vi "IMAQ FPGA Camera Link Acquisition.vi"   [LabVIEW 2017]
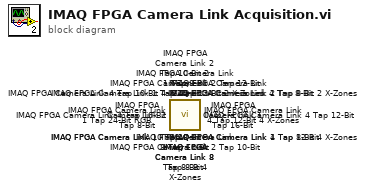
[diagram p0: block diagram]
diagram:
  n1 = call <vilib>:"IMAQ FPGA Camera Link 8 Tap 10-Bit.vi"() -> ()  [unwired: 8 in, 4 out]
  n2 = call <vilib>:"IMAQ FPGA Camera Link 2 Tap 12-Bit 2 X-Zones.vi"() -> ()  [unwired: 8 in, 4 out]
  n3 = call <vilib>:"IMAQ FPGA Camera Link 1 Tap 24-Bit RGB.vi"() -> ()  [unwired: 8 in, 4 out]
  n4 = call <vilib>:"IMAQ FPGA Camera Link 4 Tap 12-Bit 4 X-Zones.vi"() -> ()  [unwired: 8 in, 4 out]
  n5 = call <vilib>:"IMAQ FPGA Camera Link 4 Tap 10-Bit 4 X-Zones.vi"() -> ()  [unwired: 8 in, 4 out]
  n6 = call <vilib>:"IMAQ FPGA Camera Link 2 Tap 10-Bit 2 X-Zones.vi"() -> ()  [unwired: 8 in, 4 out]
  n7 = call <vilib>:"IMAQ FPGA Camera Link 8 Tap 8-Bit 4 X-Zones.vi"() -> ()  [unwired: 8 in, 4 out]
  n8 = call <vilib>:"IMAQ FPGA Camera Link 4 Tap 8-Bit 4 X-Zones.vi"() -> ()  [unwired: 8 in, 4 out]
  n9 = call <vilib>:"IMAQ FPGA Camera Link 10 Tap 8-Bit.vi"() -> ()  [unwired: 8 in, 4 out]
  n10 = call <vilib>:"IMAQ FPGA Camera Link 4 Tap 10-Bit.vi"() -> ()  [unwired: 8 in, 4 out]
  n11 = call <vilib>:"IMAQ FPGA Camera Link 4 Tap 12-Bit.vi"() -> ()  [unwired: 8 in, 4 out]
  n12 = call <vilib>:"IMAQ FPGA Camera Link 4 Tap 8-Bit.vi"() -> ()  [unwired: 8 in, 4 out]
  n13 = call <vilib>:"IMAQ FPGA Camera Link 2 Tap 12-Bit.vi"() -> ()  [unwired: 8 in, 4 out]
  n14 = call <vilib>:"IMAQ FPGA Camera Link 2 Tap 10-Bit.vi"() -> ()  [unwired: 8 in, 4 out]
  n15 = call <vilib>:"IMAQ FPGA Camera Link 2 Tap 8-Bit.vi"() -> ()  [unwired: 8 in, 4 out]
  n16 = call <vilib>:"IMAQ FPGA Camera Link 1 Tap 16-Bit.vi"() -> ()  [unwired: 8 in, 4 out]
  n17 = call <vilib>:"IMAQ FPGA Camera Link 1 Tap 14-Bit.vi"() -> ()  [unwired: 8 in, 4 out]
  n18 = call <vilib>:"IMAQ FPGA Camera Link 1 Tap 12-Bit.vi"() -> ()  [unwired: 8 in, 4 out]
  n19 = call <vilib>:"IMAQ FPGA Camera Link 1 Tap 10-Bit.vi"() -> ()  [unwired: 8 in, 4 out]
  n20 = call <vilib>:"IMAQ FPGA Camera Link 1 Tap 8-Bit.vi"() -> ()  [unwired: 8 in, 4 out]
  n21 = call <vilib>:"IMAQ FPGA Camera Link 2 Tap 8-Bit 2 X-Zones.vi"() -> ()  [unwired: 8 in, 4 out]
  n22 = call <vilib>:"IMAQ FPGA Camera Link 8 Tap 8-Bit.vi"() -> ()  [unwired: 8 in, 4 out]
